vi "Check Conditions.vi"(0 "Zone":i32, 2 "Rain Sensor":refnum<vi>, 3 "Water Pressure Sensor (%)":refnum<vi>, 5 "Step Status In":string, 7 "Zone Setup Array in":cluster{"Zone Selector":string, "Timing":dbl}[](array[cluster]), 11 "error in":errorcluster) -> (4 "Step Status Out":string, 6 "Controller Status":string, 8 "Zone Timer":dbl, 10 "Timer Status":T1=enum."Start", 15 "error out":errorcluster)   [LabVIEW 2020]
doc: "This VI check the simulation controls conditions (Rain and Water Pressure Sensor)."
uses:
  Controls/Timer Controls.ctl
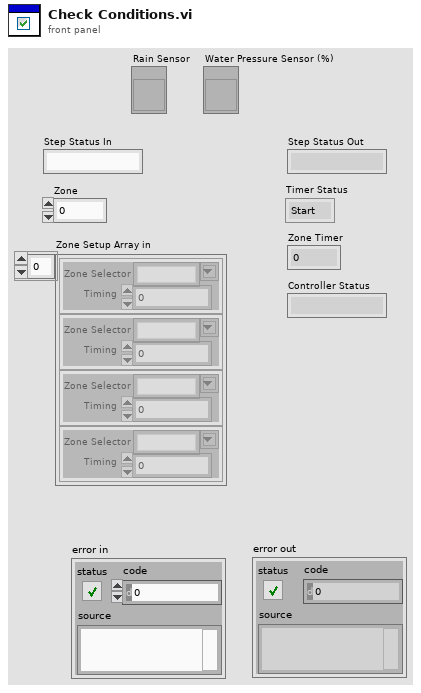
[diagram p1: front panel]
types:
  T1 = typedef "Timer Controls.ctl" = enum16{"Reset", "Start", "Stop"}
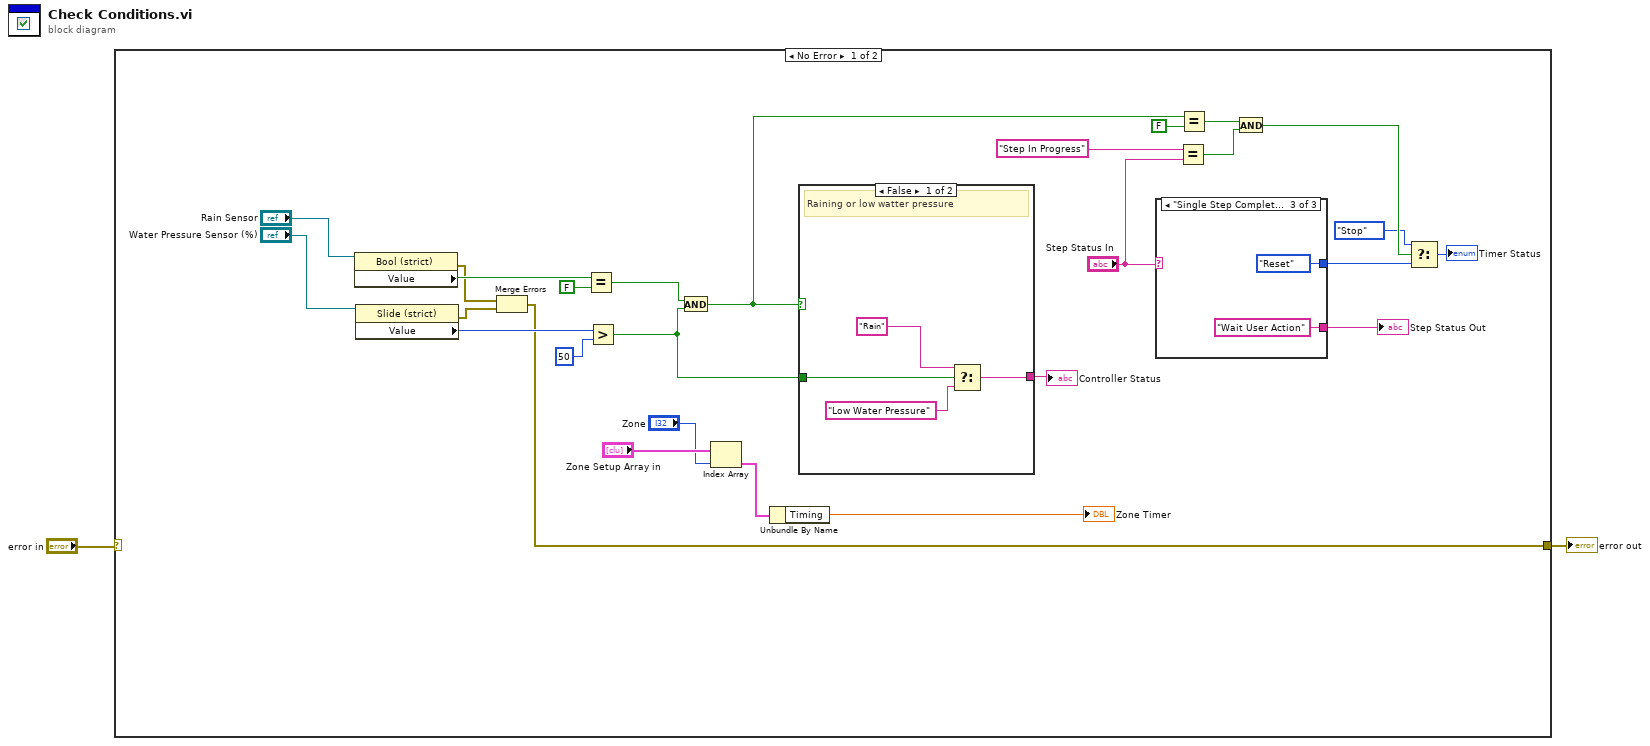
[diagram p0: block diagram]
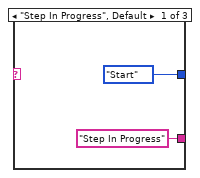
[diagram p2: hidden frame]
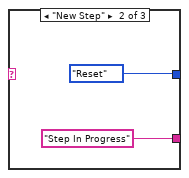
[diagram p3: hidden frame]
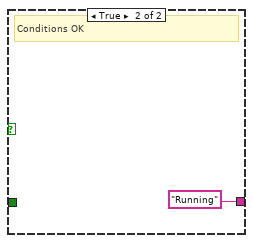
[diagram p4: hidden frame]
diagram:
  n1 = case shown="No Error" "error in" {
    selector: "error in" -> [_ w41]
    tunnel: [w14 w41] -> w1
    frame No Error {
      n2 = property class="Bool (strict)"(reference="Rain Sensor") -> (error out=w16:errorcluster, "Value"=w22:bool)  [unwired: 1 in, 1 out]
      n3 = property class="Slide (strict)"(reference="Water Pressure Sensor (%)") -> (error out=w15:errorcluster, "Value"=w24:u32)  [unwired: 1 in, 1 out]
      n4 = Merge Errors(w16, w15) -> (w14:errorcluster)
      n5 = Equal?(x=w22, y=FALSE) -> (x = y?=w20:bool)
      n6 = Greater?(x=w24, y=u32 50) -> (0:w19:bool)
      n7 = And(x=w20, y=w19) -> (x .and. y?=w7:bool)
      n8 = Index Array(array="Zone Setup Array in", index="Zone") -> (element=w26:cluster{"Zone Selector":string, "Timing":dbl})
      n9 = Unbundle By Name(w26) -> ("Timing"=→"Zone Timer":dbl)
      n10 = case shown="False" w7 {
        tunnel: [w36 "Running"] -> w18
        tunnel: w19 -> [w39 _]
        frame False {
          # "Raining or low watter pressure"
          n11 = Select(t="Rain", s=w39, f="Low Water Pressure") -> (s? t:f=w36:string)
        }
        frame True {
          # "Conditions OK"
        }
      }
      "Controller Status" <- w18
      n12 = case shown="\"Single Step Completed\"" "Step Status In" {
        tunnel: [Timer_Controls."Start" ("Timer Control") Timer_Controls."Reset" ("Timer Control") Timer_Controls."Reset" ("Timer Control")] -> w3
        tunnel: ["Step In Progress" ("Step Status 2") "Step In Progress" ("Step Status 2") "Wait User Action" ("Step Status 2")] -> w12
        frame "Step In Progress", Default {
        }
        frame "New Step" {
        }
        frame "Single Step Completed" {
        }
      }
      "Step Status Out" <- w12
      n13 = Equal?(x="Step In Progress" ("Step Status 2"), y="Step Status In") -> (x = y?=w8:bool)
      n14 = Equal?(x=w7, y=FALSE) -> (x = y?=w5:bool)
      n15 = And(x=w5, y=w8) -> (x .and. y?=w11:bool)
      n16 = Select(t=Timer_Controls."Stop" ("f"), s=w11, f=w3) -> (s? t:f=→"Timer Status":T1)
    }
    frame Error {
    }
  }
  "error out" <- w1
